vi "Drive Speed.vi"(0 "X":dbl, 2 "Y":dbl, 3 "Rotation":dbl, 5 "Enabled?":bool) -> (6 "X Out":dbl, 7 "Y Out":dbl, 8 "Rotation Out":dbl)   [LabVIEW 2014]
uses:
  <vilib>/Rock Robotics/Network Tables/SD Write Boolean.vi
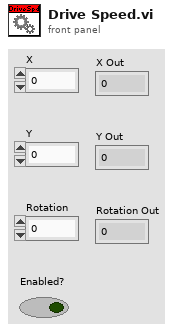
[diagram p1: front panel]
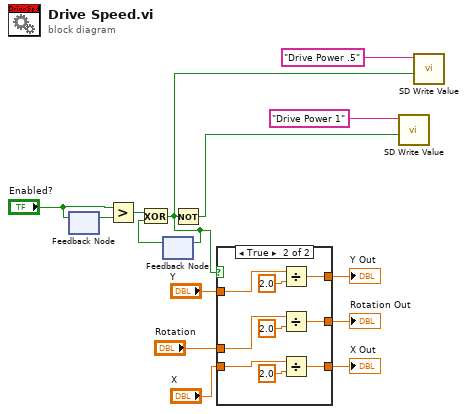
[diagram p0: block diagram]
diagram:
  n1 = feedback #1() -> (w14:bool)  [unwired: 1 in]
  n2 = feedback-in #1("Enabled?") -> ()
  n3 = Greater?(x="Enabled?", y=w14) -> (0:w13:bool)
  n4 = feedback #2() -> (w12:bool)  [unwired: 1 in]
  n5 = Exclusive Or(1:w12, 2:w13) -> (0:w4:bool)
  n6 = feedback-in #2(w4) -> ()
  n7 = Not(x=w4) -> (.not. x?=w3:bool)
  n8 = case shown="True" w4 {
    tunnel: "X" -> [w17 w26]
    tunnel: "Rotation" -> [w15 w25]
    tunnel: "Y" -> [w16 w24]
    tunnel: [w17 w18] -> w5
    tunnel: [w16 w19] -> w6
    tunnel: [w15 w20] -> w7
    frame False {
    }
    frame True {
      n9 = Divide(x=w24, y=2.0) -> (x/y=w19:dbl)
      n10 = Divide(x=w25, y=2.0) -> (x/y=w20:dbl)
      n11 = Divide(x=w26, y=2.0) -> (x/y=w18:dbl)
    }
  }
  "X Out" <- w5
  "Y Out" <- w6
  "Rotation Out" <- w7
  n12 = call-poly <vilib>:"SD Write Value.vi"("Boolean"=w3, "Name"="Drive Power 1") -> ()  [unwired: 8 in, 2 out]
  n13 = call-poly <vilib>:"SD Write Value.vi"("Boolean"=w4, "Name"="Drive Power .5") -> ()  [unwired: 8 in, 2 out]
